vi "FrisbeeIntake.vi"(0 "frisbeeIntake":enum16{"STOP", "IN", "OUT"}(ring)) -> ()   [LabVIEW 2012]
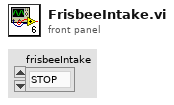
[diagram p1: front panel]
types:
  T1 = typedef "WPI_MotorControlDeviceRef.ctl" = cluster{"DeviceStatus":errorcluster, "Type":enum16{"PWM", "CAN"}, "PWM":cluster{"Digital Module":T2, "PWM Channel":T3, "DeadBand":T4}, "CAN":cluster{"Device Number":u8, "Control Mode":T5, "Semaphore":T6, "Max Vout":dbl}, "Invert":bool, "TransformRef":T7, "InvTransformRef":T7}
  T2 = typedef "FPGA_TypedefDigitalModule.ctl" = enum16{"Digital Module 1", "Digital Module 2"}
  T3 = typedef "FPGA_DIOPWMChannel.ctl" = enum8{"PWM 1", "PWM 2", "PWM 3", "PWM 4", "PWM 5", "PWM 6", "PWM 7", "PWM 8", "PWM 9", "PWM 10", "Invalid"}
  T4 = typedef "WPI_PWMDeadband.ctl" = cluster{"Name":string, "maxPositivePwm":i32, "minPositivePwm":i32, "centerPwm":i32, "maxNegativePwm":i32, "minNegativePwm":i32, "angularRange":u16}
  T5 = typedef "WPI_CANJaguar_ControlMode.ctl" = enum8{"Percent VBus", "Current", "Speed", "Position", "Voltage"}
  T6 = typedef "Semaphore RefNum" = refnum<k1>
  T7 = typedef "WPI_PWMTransform_ConPane.ctl" = refnum<vi>
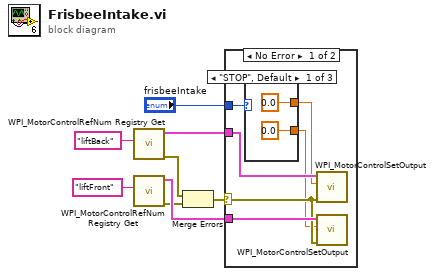
[diagram p0: block diagram]
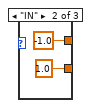
[diagram p2: hidden frame]
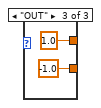
[diagram p3: hidden frame]
diagram:
  n1 = call <vilib>:"WPI_MotorControlRefNum Registry Get.vi"("refnum name"="liftBack") -> ("error out"=w3:errorcluster, "MotorControlDevRef"=w5:T1)  [unwired: 9 in]
  n2 = call <vilib>:"WPI_MotorControlRefNum Registry Get.vi"("refnum name"="liftFront") -> ("error out"=w2:errorcluster, "MotorControlDevRef"=w4:T1)  [unwired: 9 in]
  n3 = Merge Errors(w3, w2) -> (w1:errorcluster)
  n4 = case shown="No Error" w1 {
    selector: w1 -> [w11 _]
    tunnel: "frisbeeIntake" -> [w14 _]
    tunnel: w5 -> [w12 _]
    tunnel: w4 -> [w13 _]
    frame No Error {
      n5 = case shown="\"STOP\", Default" w14 {
        tunnel: [0.0 ("Output") 1.0 ("Output") -1.0 ("Output")] -> w10
        tunnel: [0.0 ("Output") -1.0 ("Output") 1.0 ("Output")] -> w9
        frame "STOP", Default {
        }
        frame "IN" {
        }
        frame "OUT" {
        }
      }
      n6 = call <vilib>:"WPI_MotorControlSetOutput.vi"("error in (no error)"=w11, "Output"=w9, "MotorControlDevRef"=w12) -> ()  [unwired: 6 in, 3 out]
      n7 = call <vilib>:"WPI_MotorControlSetOutput.vi"("error in (no error)"=w11, "Output"=w10, "MotorControlDevRef"=w13) -> ()  [unwired: 6 in, 3 out]
    }
    frame Error {
    }
  }
